vi "To JSON.vi"(5 "enable LabVIEW extensions? (T)":bool=TRUE, 6 "Pretty Print?":bool, 7 "LVClass Serializer":refnum<class "JSONtext LVClass Serializer.lvclass">, 8 "error in (no error)":errorcluster, 11 "Fake JSON Serializable in":refnum<class "Fake JSON Serializable.lvclass">) -> (0 "error out":errorcluster, 2 "<JSON>":string, 3 "Fake JSON Serializable out":refnum<class "Fake JSON Serializable.lvclass">)   [LabVIEW 2017, in "JSON Serializable Binder Tests.lvlib" / "Fake JSON Serializable.lvclass"]
doc: "Creates a JSON string from an object."
uses:
  Fake JSON Serializable.lvclass
  <vilib>/JDP Science/JSONtext/LVClass Serializer/JSONtext LVClass Serializer.lvclass
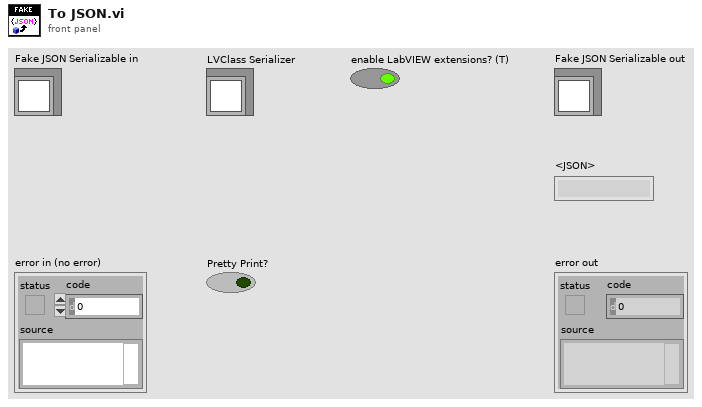
[diagram p1: front panel]
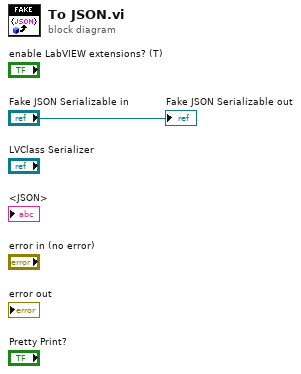
[diagram p0: block diagram]
diagram:
  "Fake JSON Serializable out" <- "Fake JSON Serializable in"
